vi "Map to SQL Insert.vi"(8 "error in (no error)":errorcluster, 10 "map in":map{string, map{string, string[]}}(c390)) -> (0 "error out":errorcluster, 2 "delimited string":string)   [LabVIEW 2019, in "LV-Data.PGSQL.lvclass"]
uses:
  LV-Data.PGSQL.lvclass
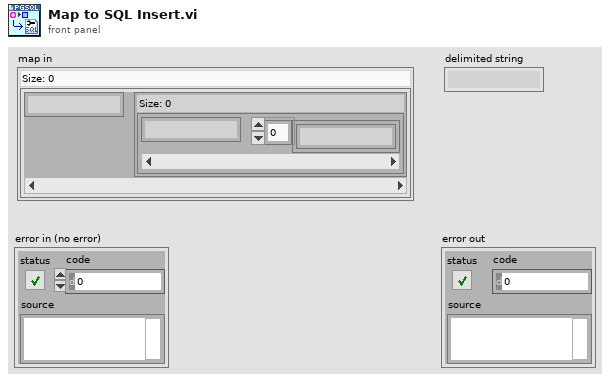
[diagram p1: front panel]
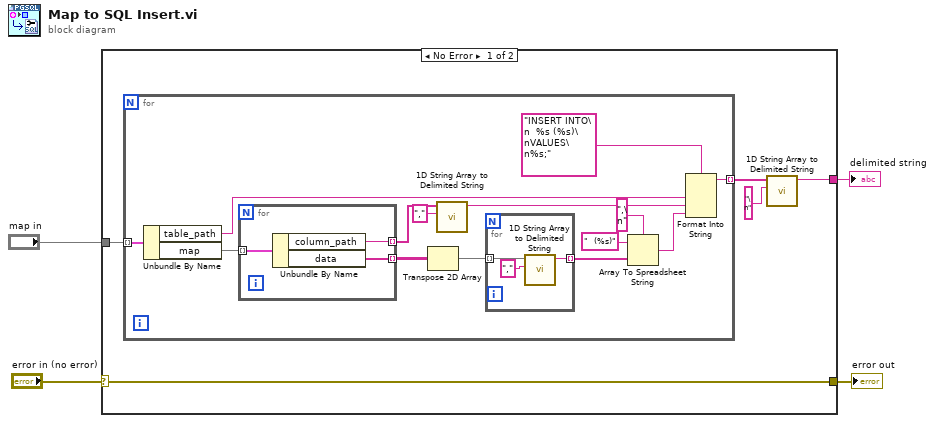
[diagram p0: block diagram]
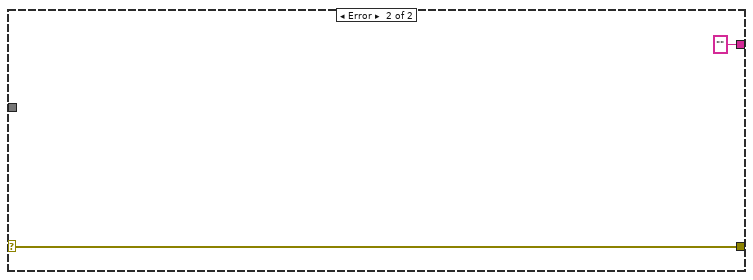
[diagram p2: hidden frame]
diagram:
  n1 = case shown="No Error" "error in (no error)" {
    selector: "error in (no error)" -> [w5 w31]
    tunnel: [w9 "" ("delimited string")] -> w4
    tunnel: "map in" -> [w6 _]
    tunnel: [w5 w31] -> w2
    frame No Error {
      n2 = for {
        tunnel: w6 -> [w23] mode=indexing
        tunnel: [w14] -> w7 mode=indexing
        n3 = Unbundle By Name(w23) -> ("table_path"=w20:string, "map"=w22:map{string, string[]})
        n4 = for {
          tunnel: w22 -> [w29] mode=indexing
          tunnel: [w28] -> w19 mode=indexing
          tunnel: [w27] -> w16 mode=indexing
          n5 = Unbundle By Name(w29) -> ("column_path"=w28:string, "data"=w27:string[])
        }
        n6 = Transpose 2D Array(2D array=w16) -> (transposed array=w15:string[][])
        n7 = call <vilib>:"1D String Array to Delimited String.vi"("delimiter"=",", "string array"=w19) -> ("delimited string"=w18:string)  [unwired: 9 in]
        n8 = for {
          tunnel: w15 -> [w26] mode=indexing
          tunnel: [w24] -> w11 mode=indexing
          n9 = call <vilib>:"1D String Array to Delimited String.vi"("delimiter"=",", "string array"=w26) -> ("delimited string"=w24:string)  [unwired: 9 in]
        }
        n10 = Array To Spreadsheet String(delimiter (Tab)=",\n", array=w11, 3:"  (%s)" ("format string")) -> (spreadsheet string=w10:string)
        n11 = Format Into String(format string="INSERT INTO\n  %s (%s)\nVALUES\n%s;", w20, w18, w10) -> (resulting string=w14:string)  [unwired: 2 in, 1 out]
      }
      n12 = call <vilib>:"1D String Array to Delimited String.vi"("delimiter"="\n", "string array"=w7) -> ("delimited string"=w9:string)  [unwired: 9 in]
    }
    frame Error {
    }
  }
  "delimited string" <- w4
  "error out" <- w2
